vi "AddSystemMappingsFromCustomDevice.vi"(7 "Add? (T)":bool=TRUE, 8 "error in":errorcluster, 10 "Frame Configuration":T1 {"CRC"."Data Type" items=["Signed", "Unsigned", "IEEE Float"]; "Rolling Counter"."Data Type" items=["Signed", "Unsigned", "IEEE Float"]; "Input Channels"."Data Type" items=["Signed", "Unsigned", "IEEE Float"]}, 11 "Node Ptr":u64 format="%.0x") -> (0 "error out":errorcluster, 2 "Frame Configuration out":T1 {"CRC"."Data Type" items=["Signed", "Unsigned", "IEEE Float"]; "Rolling Counter"."Data Type" items=["Signed", "Unsigned", "IEEE Float"]; "Input Channels"."Data Type" items=["Signed", "Unsigned", "IEEE Float"]}, 3 "Section Ref out":T4 format="%.0x")   [LabVIEW 2016, in "LIN Frame Protection Addon System Explorer.lvlib"]
uses:
  LIN Frame Protection Addon System Explorer.lvlib
  Shared/Types/FrameConfiguration.ctl
  Shared/Types/InputChannelConfiguration.ctl
  Shared/Types/Protection Type.ctl
  <vilib>/NI Veristand/Custom Device API/Custom Device Item Ref.ctl
  Shared/SubVIs/GUID Lookup.vi
  Shared/LIN Frame Protection Addon Shared.lvlib
  <vilib>/NI Veristand/Custom Device API/Custom Device API.lvlib
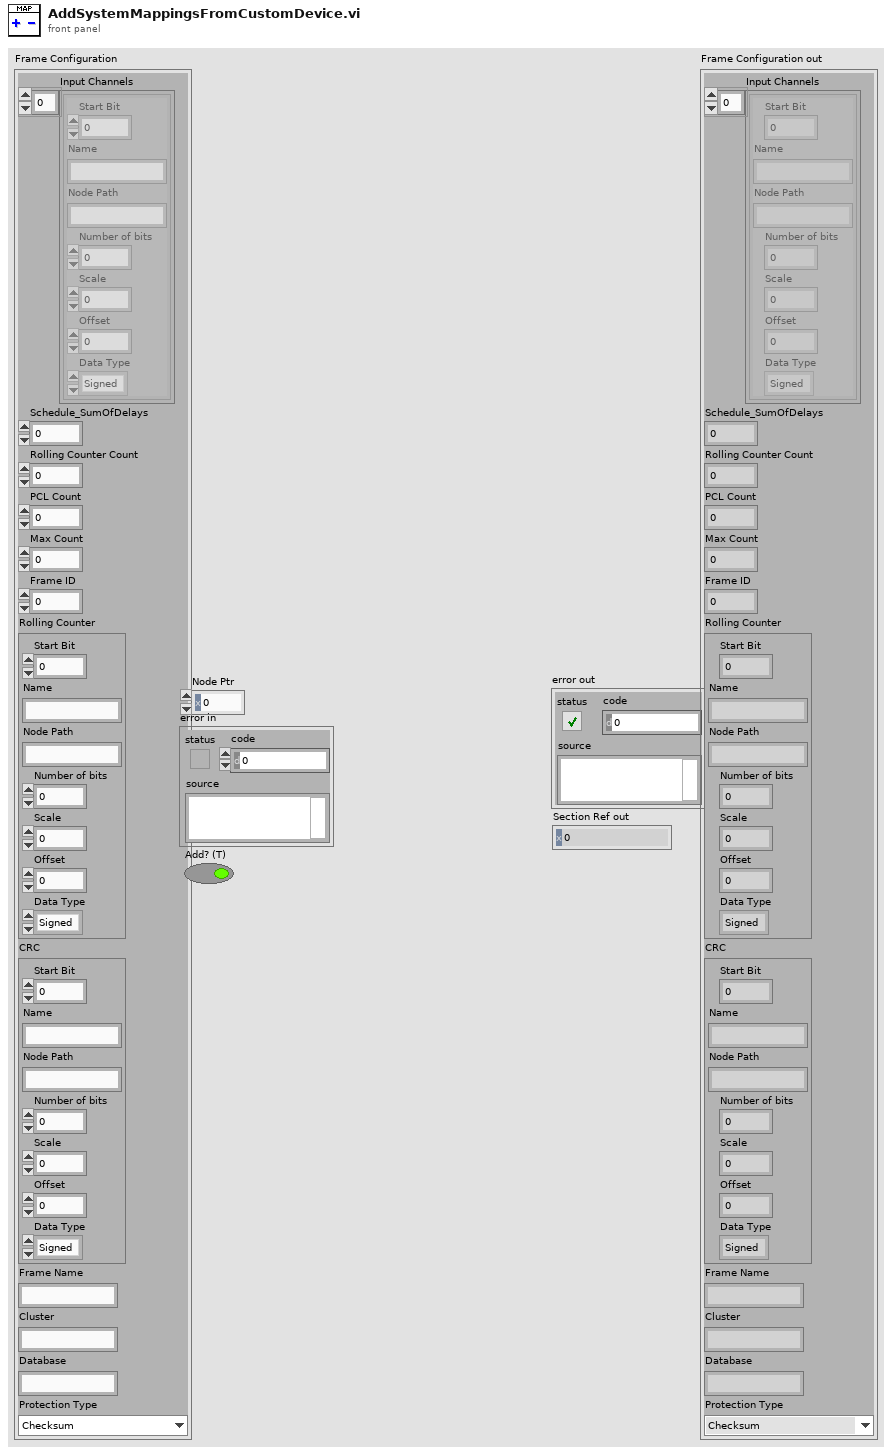
[diagram p1: front panel]
types:
  T1 = typedef "LIN Frame Protection Addon Shared.lvlib/FrameConfiguration.ctl" = cluster{"Input Channels":T2[], "Schedule_SumOfDelays":dbl, "Rolling Counter Count":dbl, "PCL Count":u64, "Max Count":dbl, "Frame ID":u32, "Rolling Counter":T2, "CRC":T2, "Frame Name":string, "Cluster":string, "Database":string, "Protection Type":T3}
  T2 = typedef "LIN Frame Protection Addon Shared.lvlib/InputChannelConfiguration.ctl" = cluster{"Start Bit":i32, "Name":string, "Node Path":string, "Number of bits":i32, "Scale":dbl, "Offset":dbl, "Data Type":u32}
  T3 = typedef "LIN Frame Protection Addon Shared.lvlib/Protection Type.ctl" = enum16{"Checksum", "CRC", "None (Counter Only)"}
  T4 = typedef "Custom Device API.lvlib/Custom Device Item Ref.ctl" = u64
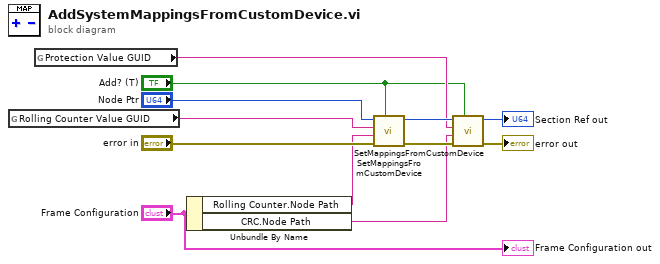
[diagram p0: block diagram]
diagram:
  n1 = global read "GUID Lookup.vi" "Rolling Counter Value GUID"() -> (w10:string)
  n2 = global read "GUID Lookup.vi" "Protection Value GUID"() -> (w5:string)
  n3 = Unbundle By Name("Frame Configuration") -> ("Rolling Counter.Node Path"=w8:string, "CRC.Node Path"=w4:string)
  n4 = call "SetMappingsFromCustomDevice.vi"("Add? (T)"="Add? (T)", "error in (no error)"="error in", "Node Path"=w8, "GUID"=w10, "Node Ptr"="Node Ptr") -> ("error out"=w7:errorcluster, "Section Ref out"=w6:T4)  [unwired: 5 in]
  n5 = call "SetMappingsFromCustomDevice.vi"("Add? (T)"="Add? (T)", "error in (no error)"=w7, "Node Path"=w4, "GUID"=w5, "Node Ptr"=w6) -> ("error out"=→"error out":errorcluster, "Section Ref out"=→"Section Ref out":T4)  [unwired: 5 in]
  "Frame Configuration out" <- "Frame Configuration"
